vi "Esophageal_ReadScore.vi"(6 "MTN Treshold":dbl=0.159 format="%#_13g", 8 "error in":errorcluster, 9 "Rep Imgs Path Location":path, 10 "Filename":string="image3_34096_18.png", 11 "HRME Scores":path) -> (0 "error out":errorcluster, 1 "HRME Score":string, 2 "Fill Color Out":u32, 3 "HRME_Score":dbl)   [LabVIEW 2021]
panel:
  in  "Command File Location":path=path "C:/Users/EsophaHRME_Dell3/Documents/GitHub/Esophageal_HRME_Software/EsophagealDeployment/Multi_Task_Network/CommandFiles/LabVIEW/cmds.json"
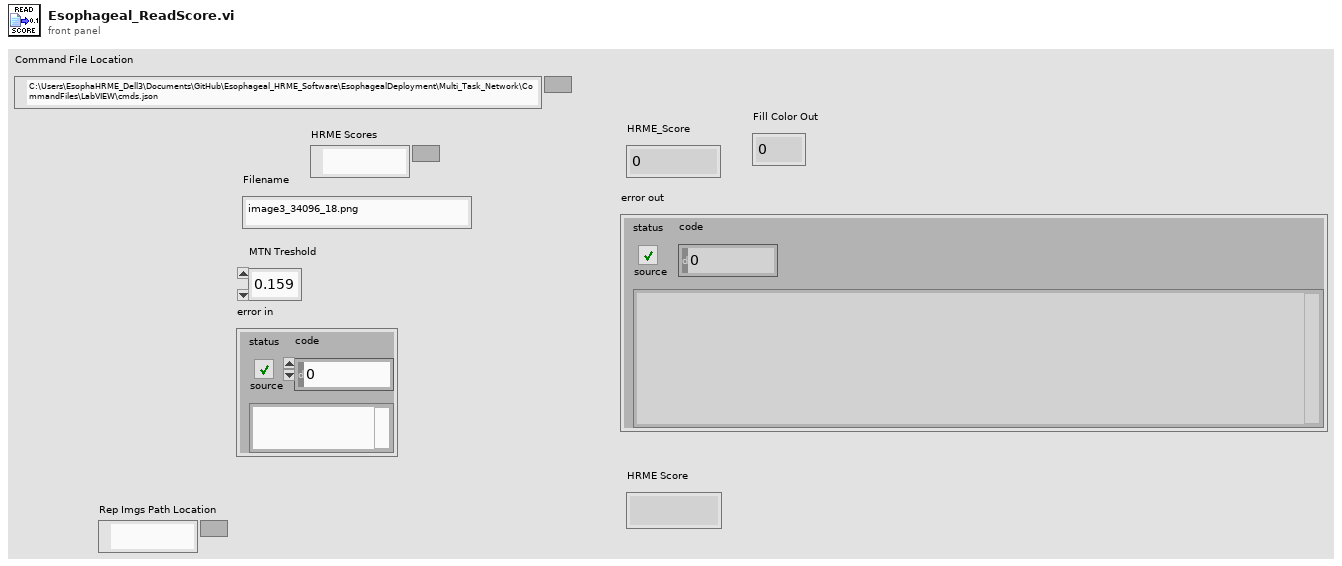
[diagram p1: front panel]
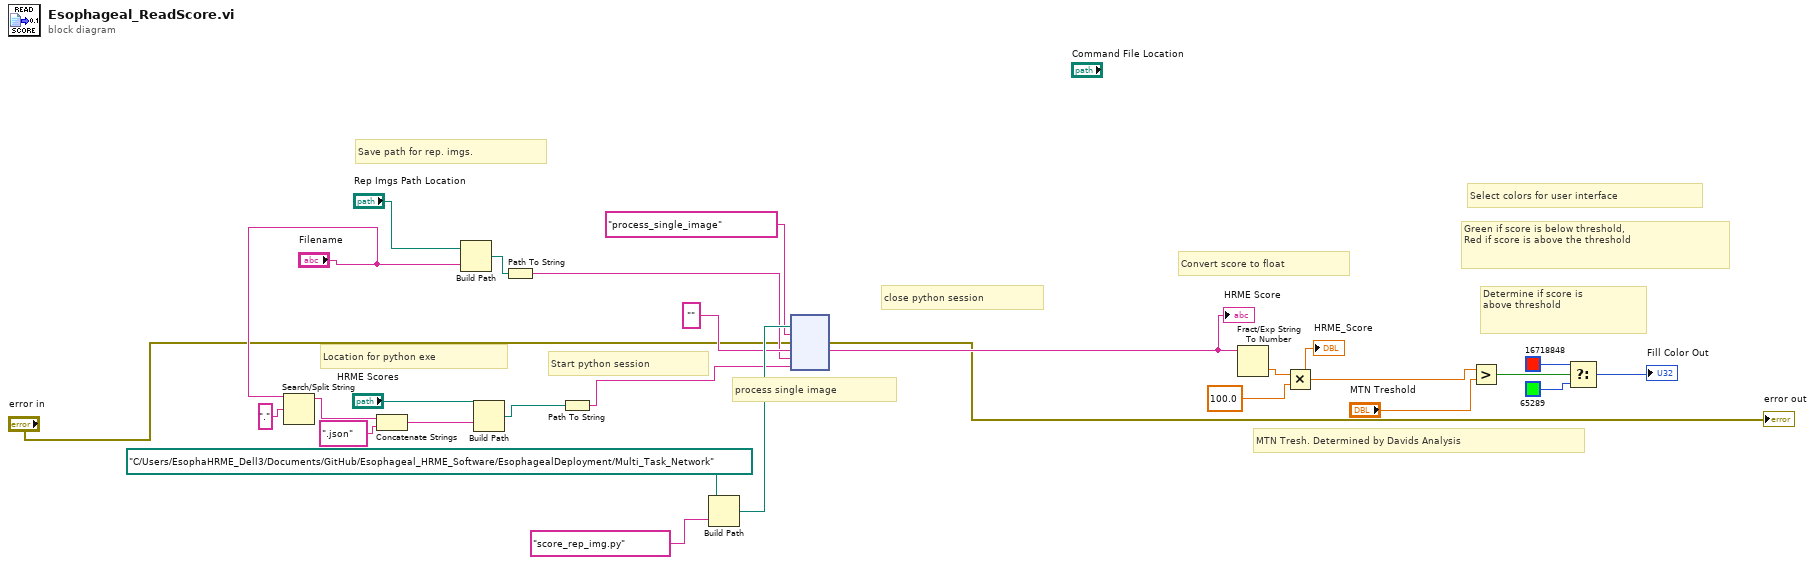
[diagram p0: block diagram]
diagram:
  # "close python session"
  # "process single image"
  # "Start python session"
  # "Location for python exe"
  # "Save path for rep. imgs."
  # "Green if score is below threshold,\nRed if score is above the threshold"
  # "Select colors for user interface"
  # "MTN Tresh. Determined by Davids Analysis"
  # "Determine if score is \nabove threshold"
  # "Convert score to float"
  n1 = Search/Split String(string="Filename", search string/char (-)=".") -> (substring before match=w7:string)  [unwired: 1 in, 2 out]
  n2 = Concatenate Strings(w7, ".json") -> (w5:string)
  n3 = Build Path(base path="Rep Imgs Path Location", name or relative path="Filename") -> (appended path=w13:path)
  n4 = Build Path(base path="HRME Scores", name or relative path=w5) -> (appended path=w4:path)
  n5 = Path To String(path=w13) -> (string=w12:string)
  n6 = Path To String(path=w4) -> (string=w3:string)
  n7 = Build Path(base path=path "C:/Users/EsophaHRME_Dell3/Documents/GitHub/Esophageal_HRME_Software/EsophagealDeployment/Multi_Task_Network", name or relative path="score_rep_img.py") -> (appended path=w17:path)
  n8 = node(w17, "process_single_image", "error in", "", w12, w3) -> (→"error out":errorcluster, w14:string)  [unwired: 3 in, 3 out]
  "HRME Score" <- w14
  n9 = Fract/Exp String To Number(string=w14) -> (number=w21:dbl)  [unwired: 3 in, 1 out]
  n10 = Multiply(x=w21, y=100.0) -> (x*y=w20:dbl)
  "HRME_Score" <- w20
  n11 = Greater?(x=w20, y="MTN Treshold") -> (0:w26:bool)
  n12 = Select(t=u32 16718848, s=w26, f=u32 65289) -> (s? t:f=→"Fill Color Out":u32)
